vi "Compile Engine Data.vi"(8 "error in (no error)":errorcluster, 11 "Device Item Ref in":T1 format="%.0x") -> (0 "error out":errorcluster)   [LabVIEW 2017, in "NI 272x Resistive Simulation Custom Device Configuration.lvlib"]
uses:
  NI 272x Resistive Simulation Custom Device Configuration.lvlib
  <vilib>/NI Veristand/Custom Device API/Custom Device Item Ref.ctl
  Controls/Compiled Engine Data.ctl
  Controls/Compiled HW Channel.ctl
  Controls/Channel Mode.ctl
  <instrlib>/ni272xReferenceVIs/ni272xReferenceVIs.llb/ni272x Callendar-Van Dusen RTD Parameters.ctl
  Controls/Compiled Connect Channel.ctl
  Globals/Names.vi
  <vilib>/NI Veristand/Custom Device API/Get Item Property (String).vi
  <vilib>/NI Veristand/Custom Device API/Get Item Property (Double).vi
  <vilib>/NI Veristand/Custom Device API/Set Item Property (Variant).vi
  NI 272x Resistive Simulation Custom Device Shared.lvlib
  <vilib>/NI VeriStand/Custom Device API/Custom Device API.lvlib
  <vilib>/NI/NIVS Inline Async API/_Data Access System Explorer/Data Access System Explorer.lvlib
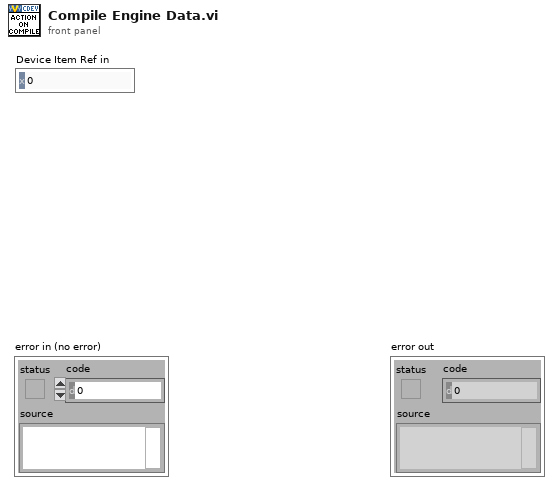
[diagram p1: front panel]
types:
  T1 = typedef "Custom Device API.lvlib/Custom Device Item Ref.ctl" = u64
  T2 = typedef "NI 272x Resistive Simulation Custom Device Shared.lvlib/Compiled Engine Data.ctl" = cluster{"HW Chns":T3[], "Con Chns":T6[], "DevName":string, "TL dt":i64}
  T3 = typedef "NI 272x Resistive Simulation Custom Device Shared.lvlib/Compiled HW Channel.ctl" = cluster{"Mode":T4, "RTD":T5, "Last Des Val":dbl, "HW CH":string}
  T4 = typedef "NI 272x Resistive Simulation Custom Device Shared.lvlib/Channel Mode.ctl" = enum16{"Resistance", "RTD Temperature"}
  T5 = typedef "ni272x Callendar-Van Dusen RTD Parameters.ctl" = cluster{"A":dbl, "B":dbl, "C":dbl, "R0":dbl}
  T6 = typedef "NI 272x Resistive Simulation Custom Device Shared.lvlib/Compiled Connect Channel.ctl" = cluster{"HW CH":string, "Is Con":bool, "HW CH+1":string}
  T7 = cluster{"Name":string, "Type":enum16{"Output/Write", "Input/Read", "Input/ReadWrite"}, "VS Refs":T1[]}
  T8 = cluster{"Name":string, "Type":enum16{"Output/Write", "Input/Read", "Input/ReadWrite"}, "VS Refs":T1[]}[]
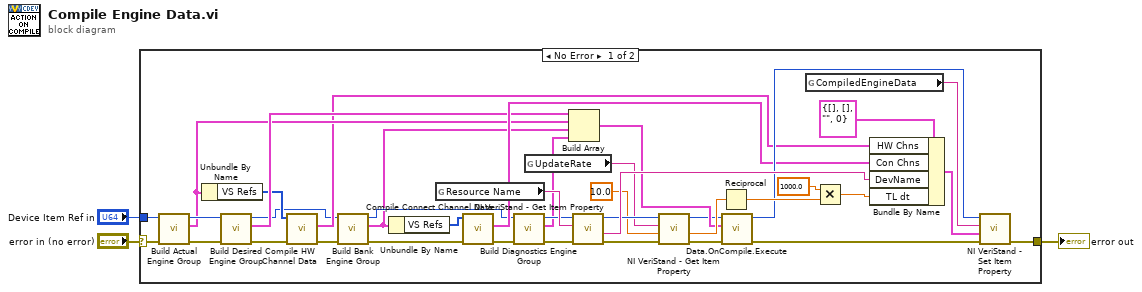
[diagram p0: block diagram]
diagram:
  n1 = case shown="No Error" "error in (no error)" {
    selector: "error in (no error)" -> [w42 w43]
    tunnel: [w35 w43] -> w2
    tunnel: "Device Item Ref in" -> [w22 _]
    frame No Error {
      n2 = call "Build Actual Engine Group.vi"("error in (no error)"=w42, "Device Item Ref in"=w22) -> ("error out"=w21:errorcluster, "Group"=w9:T7, "Section Ref out"=w20:T1)  [unwired: 7 in]
      n3 = Unbundle By Name(w9) -> ("VS Refs"=w7:T1[])
      n4 = call "Build Desired Engine Group.vi"("error in (no error)"=w21, "Section Ref in"=w20) -> ("error out"=w41:errorcluster, "Group"=w13:T7, "Section Ref out"=w4:T1)  [unwired: 7 in]
      n5 = call "Compile HW Channel Data.vi"("error in (no error)"=w41, "Desired Values Refs"=w7) -> ("error out"=w39:errorcluster, "Compiled HW Channels"=w6:T3[])  [unwired: 8 in]
      n6 = call "Build Bank Engine Group.vi"("error in (no error)"=w39, "Device ref dup"=w4) -> ("error out"=w38:errorcluster, "Group"=w8:T7, "Section Ref out"=w12:T1)  [unwired: 7 in]
      n7 = Unbundle By Name(w8) -> ("VS Refs"=w5:T1[])
      n8 = global read "Names.vi" "Resource Name"() -> (w31:string)
      n9 = call "Compile Connect Channel Data.vi"("error in (no error)"=w38, "Connect Chan Refs"=w5) -> ("error out"=w37:errorcluster, "Compiled HW Channels"=w14:T6[])  [unwired: 8 in]
      n10 = call "Build Diagnostics Engine Group.vi"("error in (no error)"=w37, "Section Ref in"=w12) -> ("error out"=w36:errorcluster, "Group"=w10:T7, "Section Ref out"=w11:T1)  [unwired: 7 in]
      n11 = global read "Names.vi" "UpdateRate"() -> (w28:string)
      n12 = Build Array(w13, w9, w8, w10) -> (w19:T8)
      n13 = call-poly <vilib>:"NI VeriStand - Get Item Property.vi"("error in (no error)"=w36, "Property Name"=w31, "Item Ref in"=w11) -> ("error out"=w32:errorcluster, "Value"=w30:string, "Item Ref out"=w29:T1)  [unwired: 5 in, 1 out]
      n14 = call-poly <vilib>:"NI VeriStand - Get Item Property.vi"("error in (no error)"=w32, "Default Value"=10.0, "Property Name"=w28, "Item Ref in"=w29) -> ("error out"=w16:errorcluster, "Value"=w24:dbl, "Item Ref out"=w18:T1)  [unwired: 4 in, 1 out]
      n15 = Reciprocal(x=w24) -> (1/x=w26:dbl)
      n16 = call <vilib>:"Data.OnCompile.Execute.vi"("error in"=w16, "VS Ref Groups"=w19, "Custom Device Ref"=w18) -> ("error out"=w15:errorcluster, "Custom Device Ref"=w17:T1)  [unwired: 7 in]
      n17 = global read "Names.vi" "CompiledEngineData"() -> (w34:string)
      n18 = Multiply(x=1000.0, y=w26) -> (x*y=w23:dbl)
      n19 = Bundle By Name(cluster=T2 {"HW Chns"=[], "Con Chns"=[], "DevName"="", "TL dt"=0} ("Engine Run Time Data"), "HW Chns"=w6, "Con Chns"=w14, "DevName"=w30, "TL dt"=w23) -> (w33:T2)
      n20 = call-poly <vilib>:"NI VeriStand - Set Item Property.vi"("error in (no error)"=w15, "Value"=w33, "Property Name"=w34, "Item Ref in"=w17) -> ("error out"=w35:errorcluster)  [unwired: 5 in, 2 out]
    }
    frame Error {
    }
  }
  "error out" <- w2
